vi "Arrange Horizontal.vi"(8 "error in (no error)":errorcluster, 11 "[MDI] Parent in":refnum<class "[MDI] Parent.lvclass">) -> (0 "error out":errorcluster, 3 "[MDI] Parent out":refnum<class "[MDI] Parent.lvclass">)   [LabVIEW 2020, in "[MDI] Parent.lvlib" / "[MDI] Parent.lvclass"]
uses:
  [MDI] Parent.lvclass
  [MDI] Parent.lvclass/[MDI] Parent.ctl
panel:
  out "error":u32
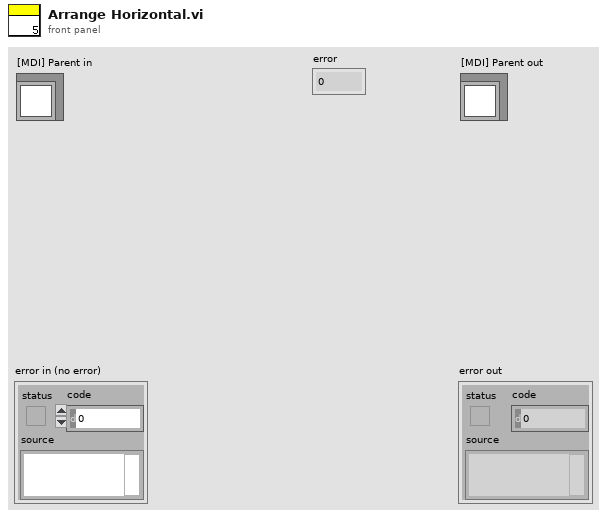
[diagram p1: front panel]
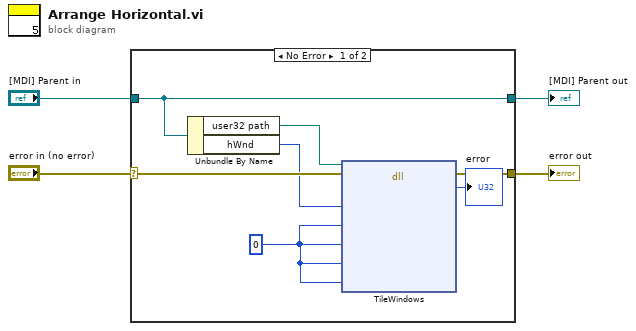
[diagram p0: block diagram]
diagram:
  n1 = case shown="No Error" "error in (no error)" {
    selector: "error in (no error)" -> [w10 w13]
    tunnel: [w9 w13] -> w3
    tunnel: [w11 w12] -> w1
    tunnel: "[MDI] Parent in" -> [w11 w12]
    frame No Error {
      w7 = u32 0 ("wHow")
      n2 = Unbundle By Name(w11) -> ("user32 path"=w6:path, "hWnd"=w8:u32)
      n3 = dll-call lib="user32.dll" fn="TileWindows"(path in=w6, error in=w10, "hWndParent"=w8, "wHow"=w7, "rect"=w7, "cKids"=w7, "IpKids"=w7) -> (error out=w9:errorcluster, "error"=→"error":u32)  [unwired: 6 in, 1 out]
    }
    frame Error {
    }
  }
  "error out" <- w3
  "[MDI] Parent out" <- w1
